vi "Replace Item at Offset.vi"(8 "error in (no error)":errorcluster, 9 "New JSON Item":string, 10 "Offset of Item to Replace":i32, 11 "JSON":string) -> (0 "error out":errorcluster, 3 "<JSON>":string)   [LabVIEW 2021, in "json.facade.lvlib"]
doc: "Replace the JSON Value located at an Offset in the input JSON. The Offset can be that returned by a previous \"Find\" operation on the input JSON."
uses:
  json.facade.lvlib
  jsontext/JSONtext.lvlib
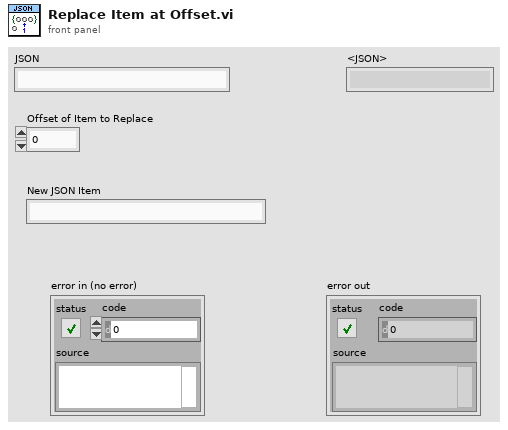
[diagram p1: front panel]
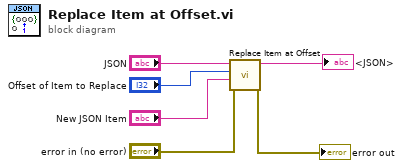
[diagram p0: block diagram]
diagram:
  n1 = call "Replace Item at Offset.vi"("error in (no error)"="error in (no error)", "New JSON Item"="New JSON Item", "Offset of Item to Replace"="Offset of Item to Replace", "JSON"="JSON") -> ("error out"=→"error out":errorcluster, "<JSON>"=→"<JSON>":string)  [unwired: 6 in]
